vi "Next Capture.vi"(8 "error in (no error)":errorcluster, 9 "timeout (ms)":u16, 10 "ARGB Image Destination":refnum<data-value>, 11 "CameraStream in":refnum<class "CameraStream.lvclass">) -> (0 "error out":errorcluster, 2 "ARGB Image (duplicate)":refnum<data-value>, 3 "CameraStream (Duplicate)":refnum<class "CameraStream.lvclass">)   [LabVIEW 2020, in "g_ar_toolkit.capture.lvlib" / "CameraStream.lvclass"]
uses:
  CameraStream.lvclass
  CameraStream.lvclass/CameraStream.ctl
  g_ar_toolkit.common/g_ar_toolkit.common.lvlib
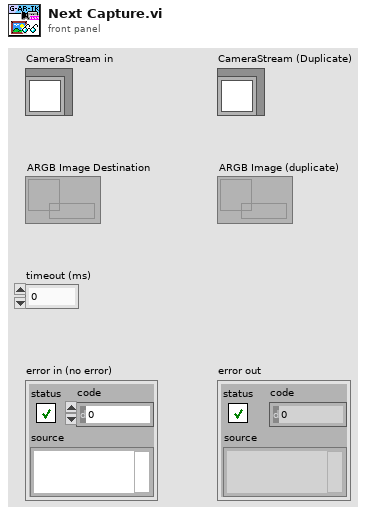
[diagram p1: front panel]
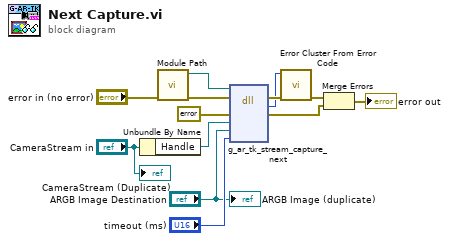
[diagram p0: block diagram]
diagram:
  n1 = Unbundle By Name("CameraStream in") -> ("Handle"=w10:refnum<data-value>)
  n2 = call "Module Path.vi"("error in (no error)"="error in (no error)") -> ("error out"=w2:errorcluster, "Path"=w1:path)  [unwired: 9 in]
  n3 = dll-call lib="?" fn="g_ar_tk_stream_capture_next"(path in=w1, error in=w2, "error_cluster"=errorcluster {"status"=FALSE, "code"=0, "source"=""} ("error constant"), "EDVR_strm"=w10, "EDVR_img"="ARGB Image Destination", "timeout"="timeout (ms)") -> (error out=w8:errorcluster, "MgErr"=w7:i32, "error_cluster"=w5:errorcluster)  [unwired: 4 in, 1 out]
  n4 = call <vilib>:"Error Cluster From Error Code.vi"("error in (no error)"=w8, "error code (0)"=w7) -> ("error out"=w6:errorcluster)  [unwired: 7 in]
  n5 = Merge Errors(w6, w5) -> (→"error out":errorcluster)
  "CameraStream (Duplicate)" <- "CameraStream in"
  "ARGB Image (duplicate)" <- "ARGB Image Destination"
